vi "界面参数读取.vi"(1 "路径":path=path "E:/LabVIEW/福尔达/AppData") -> (0 "标准":T1)   [LabVIEW 2018]
uses:
  <vilib>/Utility/config.llb/Read Key (String).vi
  <vilib>/Utility/config.llb/NI_LVConfig.lvlib
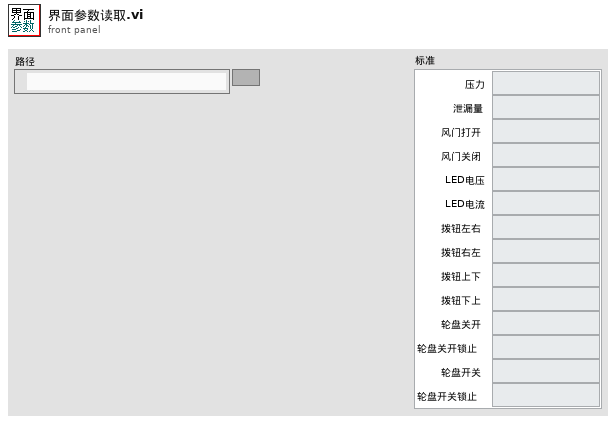
[diagram p1: front panel]
types:
  T1 = cluster{"压力":string, "泄漏量":string, "风门打开":string, "风门关闭":string, "LED电压":string, "LED电流":string, "拨钮左右":string, "拨钮右左":string, "拨钮上下":string, "拨钮下上":string, "轮盘关开":string, "轮盘关开锁止":string, "轮盘开关":string, "轮盘开关锁止":string}
  T2 = typedef "NI_LVConfig.lvlib/Config Data RefNum.ctl" = refnum<k1>
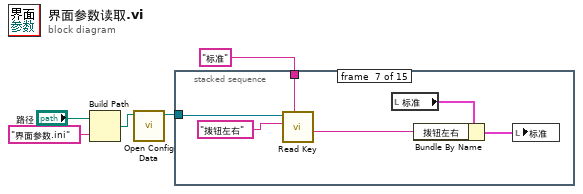
[diagram p0: block diagram]
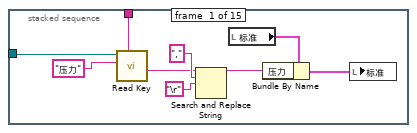
[diagram p2: hidden frame]
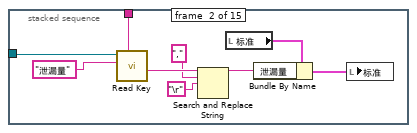
[diagram p3: hidden frame]
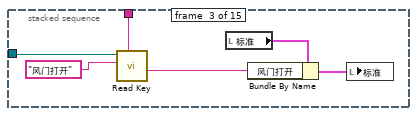
[diagram p4: hidden frame]
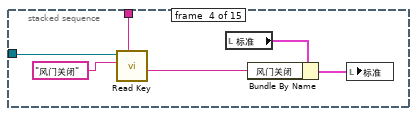
[diagram p5: hidden frame]
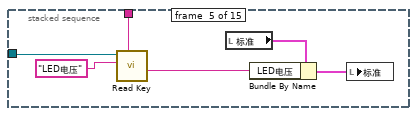
[diagram p6: hidden frame]
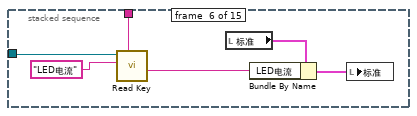
[diagram p7: hidden frame]
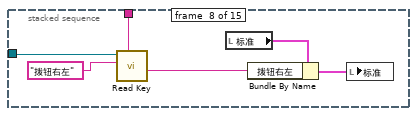
[diagram p8: hidden frame]
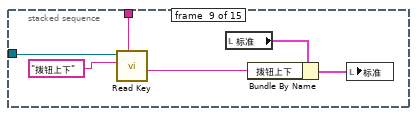
[diagram p9: hidden frame]
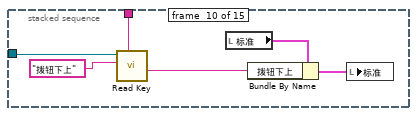
[diagram p10: hidden frame]
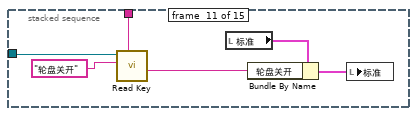
[diagram p11: hidden frame]
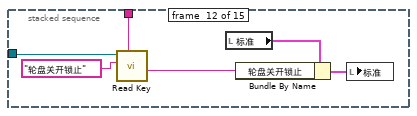
[diagram p12: hidden frame]
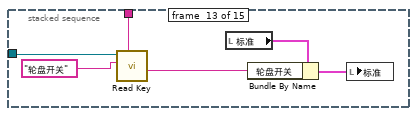
[diagram p13: hidden frame]
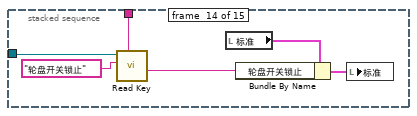
[diagram p14: hidden frame]
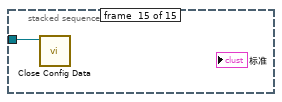
[diagram p15: hidden frame]
diagram:
  n1 = Build Path(base path="路径", name or relative path="界面参数.ini" ("名称或相对路径")) -> (appended path=w3:path)
  n2 = call <vilib>:"Open Config Data.vi"("configuration file path"=w3) -> ("refnum"=w2:T2)  [unwired: 8 in, 2 out]
  n3 = stacked-sequence {
    tunnel: w2 -> [w14 w23 w29 w35 w41 w47 w53 w59 w65 w71 w77 w83 w89 w95 w96]
    tunnel: "标准" -> [w13 w22 w28 w34 w40 w46 w52 w58 w64 w70 w76 w82 w88 w94 _]
    frame #0 {
      n4 = call-poly <vilib>:"Read Key.vi"("section"=w13, "key"="压力", "refnum"=w14) -> ("value"=w7:string)  [unwired: 5 in, 3 out]
      n5 = Search and Replace String(input string=w7, search string="," ("搜索字符串"), replace string="\r") -> (result string=w6:string)  [unwired: 5 in, 3 out]
      n6 = local read "标准"() -> (w12:T1)
      n7 = Bundle By Name(cluster=w12, "压力"=w6) -> (w11:T1)
      n8 = local write "标准"(w11) -> ()
    }
    frame #1 {
      n9 = call-poly <vilib>:"Read Key.vi"("section"=w22, "key"="泄漏量", "refnum"=w23) -> ("value"=w18:string)  [unwired: 5 in, 3 out]
      n10 = Search and Replace String(input string=w18, search string="," ("搜索字符串"), replace string="\r") -> (result string=w15:string)  [unwired: 5 in, 3 out]
      n11 = local read "标准"() -> (w21:T1)
      n12 = Bundle By Name(cluster=w21, "泄漏量"=w15) -> (w20:T1)
      n13 = local write "标准"(w20) -> ()
    }
    frame #2 {
      n14 = call-poly <vilib>:"Read Key.vi"("section"=w28, "key"="风门打开", "refnum"=w29) -> ("value"=w24:string)  [unwired: 5 in, 3 out]
      n15 = local read "标准"() -> (w27:T1)
      n16 = Bundle By Name(cluster=w27, "风门打开"=w24) -> (w26:T1)
      n17 = local write "标准"(w26) -> ()
    }
    frame #3 {
      n18 = call-poly <vilib>:"Read Key.vi"("section"=w34, "key"="风门关闭", "refnum"=w35) -> ("value"=w31:string)  [unwired: 5 in, 3 out]
      n19 = local read "标准"() -> (w33:T1)
      n20 = Bundle By Name(cluster=w33, "风门关闭"=w31) -> (w32:T1)
      n21 = local write "标准"(w32) -> ()
    }
    frame #4 {
      n22 = call-poly <vilib>:"Read Key.vi"("section"=w40, "key"="LED电压", "refnum"=w41) -> ("value"=w37:string)  [unwired: 5 in, 3 out]
      n23 = local read "标准"() -> (w39:T1)
      n24 = Bundle By Name(cluster=w39, "LED电压"=w37) -> (w38:T1)
      n25 = local write "标准"(w38) -> ()
    }
    frame #5 {
      n26 = call-poly <vilib>:"Read Key.vi"("section"=w46, "key"="LED电流", "refnum"=w47) -> ("value"=w43:string)  [unwired: 5 in, 3 out]
      n27 = local read "标准"() -> (w45:T1)
      n28 = Bundle By Name(cluster=w45, "LED电流"=w43) -> (w44:T1)
      n29 = local write "标准"(w44) -> ()
    }
    frame #6 {
      n30 = call-poly <vilib>:"Read Key.vi"("section"=w52, "key"="拨钮左右", "refnum"=w53) -> ("value"=w49:string)  [unwired: 5 in, 3 out]
      n31 = local read "标准"() -> (w51:T1)
      n32 = Bundle By Name(cluster=w51, "拨钮左右"=w49) -> (w50:T1)
      n33 = local write "标准"(w50) -> ()
    }
    frame #7 {
      n34 = call-poly <vilib>:"Read Key.vi"("section"=w58, "key"="拨钮右左", "refnum"=w59) -> ("value"=w55:string)  [unwired: 5 in, 3 out]
      n35 = local read "标准"() -> (w57:T1)
      n36 = Bundle By Name(cluster=w57, "拨钮右左"=w55) -> (w56:T1)
      n37 = local write "标准"(w56) -> ()
    }
    frame #8 {
      n38 = call-poly <vilib>:"Read Key.vi"("section"=w64, "key"="拨钮上下", "refnum"=w65) -> ("value"=w61:string)  [unwired: 5 in, 3 out]
      n39 = local read "标准"() -> (w63:T1)
      n40 = Bundle By Name(cluster=w63, "拨钮上下"=w61) -> (w62:T1)
      n41 = local write "标准"(w62) -> ()
    }
    frame #9 {
      n42 = call-poly <vilib>:"Read Key.vi"("section"=w70, "key"="拨钮下上", "refnum"=w71) -> ("value"=w67:string)  [unwired: 5 in, 3 out]
      n43 = local read "标准"() -> (w69:T1)
      n44 = Bundle By Name(cluster=w69, "拨钮下上"=w67) -> (w68:T1)
      n45 = local write "标准"(w68) -> ()
    }
    frame #10 {
      n46 = call-poly <vilib>:"Read Key.vi"("section"=w76, "key"="轮盘关开", "refnum"=w77) -> ("value"=w73:string)  [unwired: 5 in, 3 out]
      n47 = local read "标准"() -> (w75:T1)
      n48 = Bundle By Name(cluster=w75, "轮盘关开"=w73) -> (w74:T1)
      n49 = local write "标准"(w74) -> ()
    }
    frame #11 {
      n50 = call-poly <vilib>:"Read Key.vi"("section"=w82, "key"="轮盘关开锁止", "refnum"=w83) -> ("value"=w79:string)  [unwired: 5 in, 3 out]
      n51 = local read "标准"() -> (w81:T1)
      n52 = Bundle By Name(cluster=w81, "轮盘关开锁止"=w79) -> (w80:T1)
      n53 = local write "标准"(w80) -> ()
    }
    frame #12 {
      n54 = call-poly <vilib>:"Read Key.vi"("section"=w88, "key"="轮盘开关", "refnum"=w89) -> ("value"=w85:string)  [unwired: 5 in, 3 out]
      n55 = local read "标准"() -> (w87:T1)
      n56 = Bundle By Name(cluster=w87, "轮盘开关"=w85) -> (w86:T1)
      n57 = local write "标准"(w86) -> ()
    }
    frame #13 {
      n58 = call-poly <vilib>:"Read Key.vi"("section"=w94, "key"="轮盘开关锁止", "refnum"=w95) -> ("value"=w91:string)  [unwired: 5 in, 3 out]
      n59 = local read "标准"() -> (w93:T1)
      n60 = Bundle By Name(cluster=w93, "轮盘开关锁止"=w91) -> (w92:T1)
      n61 = local write "标准"(w92) -> ()
    }
    frame #14 {
      n62 = call <vilib>:"Close Config Data.vi"("refnum"=w96) -> ()  [unwired: 9 in, 2 out]
    }
  }
